vi "FRC3005_GyroXRS450_SPI_Accumulator_Loop.vi"(8 "error in":errorcluster, 10 "History Length (ms)":i32=2000, 11 "GyroDeviceRef":T1={"DevStatus"={"status"=FALSE, "code"=0, "source"=""}, "Analog Channel"=enum."AI 0", "Offset"=0.0, "Gain (VoltsPerDegree/Second)"=0.0, "Gyro Type"=enum."Analog", "Handle"=0, "SPI Bus"=enum."Invalid", "Device Found"=FALSE, "Sample Rate"=1.0, "Calibrate On Open"=FALSE} {"Sample Rate" min=0.25 max=100.0 step=0.25}) -> (0 "error out":errorcluster)   [LabVIEW 2016, in "Path Track.lvlib"]
doc: "Periodically reads the SimpleGyro and makes data available to your robot project. Place this block within PeriodicTasks.vi."
uses:
  Path Track.lvlib
  <vilib>/Rock Robotics/WPI/Gyro/WPI_GyroDevRef.ctl
  <vilib>/Rock Robotics/SystemInterfaces/AI/FPGA_AIChannel.ctl
  <vilib>/Rock Robotics/SystemInterfaces/spilib/spi_bus.ctl
  <vilib>/Rock Robotics/WPI/SPI/WPI_SPIDevRef.ctl
  FGV Control.ctl
  <vilib>/Platform/TimedLoop/XDataNode/timing_clust.ctl
  <vilib>/Platform/TimedLoop/XDataNode/nitl_modes.ctl
  <vilib>/Platform/TimedLoop/XDataNode/wakeup.ctl
  <vilib>/Platform/TimedLoop/XDataNode/XDataNode.xnode
  <vilib>/Platform/TimedLoop/XDataNode/XDNodeRunTimeDep.lvlib
  <vilib>/ptbypt/NI_PtbyPt.lvlib
panel:
  out "Rate":dbl
  out "Device Found":bool
  out "Offset":dbl
  out "Angle":dbl
  # "Analog"
  # "XRS"
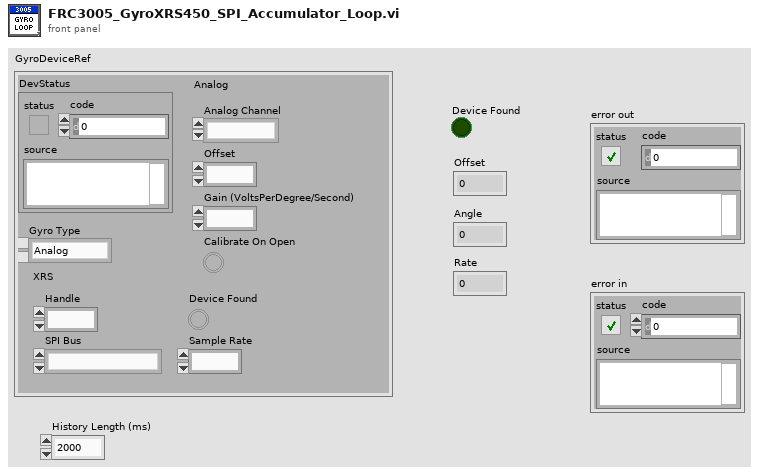
[diagram p1: front panel]
types:
  T1 = typedef "WPI_GyroDevRef.ctl" = cluster{"DevStatus":errorcluster, "Analog Channel":T2, "Offset":dbl, "Gain (VoltsPerDegree/Second)":dbl, "Gyro Type":enum16{"Analog", "XRS450"}, "Handle":i32, "SPI Bus":T3, "Device Found":bool, "Sample Rate":dbl, "Calibrate On Open":bool}
  T2 = typedef "FPGA_AIChannel.ctl" = enum8{"AI 0", "AI 1", "AI 2", "AI 3", "AI MXP 0", "AI MXP 1", "AI MXP 2", "AI MXP 3", "Invalid"}
  T3 = typedef "spi_bus.ctl" = enum16{"SPI On-Board, CS0", "SPI On-Board, CS1", "SPI On-Board, CS2", "SPI On-Board, CS3", "SPI MXP", "Invalid"}
  T4 = typedef "WPI_SPIDevRef.ctl" = cluster{"DevStatus":errorcluster, "Handle":i32, "SPI Bus":T3}
  T5 = typedef "Path Track.lvlib/FGV Control.ctl" = enum16{"Allocate", "Get", "Append"}
  T6 = typedef "XDNodeRunTimeDep.lvlib/timing_clust.ctl" = cluster{"Expected End [f-1]":u64, "Actual End [f-1]":u64, "Finished Late? [f-1]":bool, "Expected End [i-1]":u64, "Actual End [i-1]":u64, "Finished Late? [i-1]":bool, "Expected Start [i]":u64, "Actual Start [i]":u64, "Expected Start [f]":u64, "Actual Start [f]":u64, "Source Name":string, "Structure Name":string, "Period":i64, "Deadline":i64, "Offset":i64, "Start":i64, "Priority":i32, "Timeout":i32, "Mode":T7, "Wakeup Reason":T8, "Error":errorcluster, "Source Type":string, "Secondary Source Type":string, "Global End Time":u64, "Global Start Time":u64, "Frame Duration":u64, "Iteration Duration":u64, "Assigned CPU":i32, "I/O Scan Engine Mode":u32}
  T7 = typedef "XDNodeRunTimeDep.lvlib/nitl_modes.ctl" = enum32{"No Change", "Process missed periods, maintain original phase", "Discard missed periods, maintain original phase", "Process missed periods, ignore original phase", "Discard missed periods, ignore original phase"}
  T8 = typedef "XDNodeRunTimeDep.lvlib/wakeup.ctl" = enum32{"Normal", "Aborted", "Asynchronous wakeup", "Timing source error", "Timed loop error", "Timeout"}
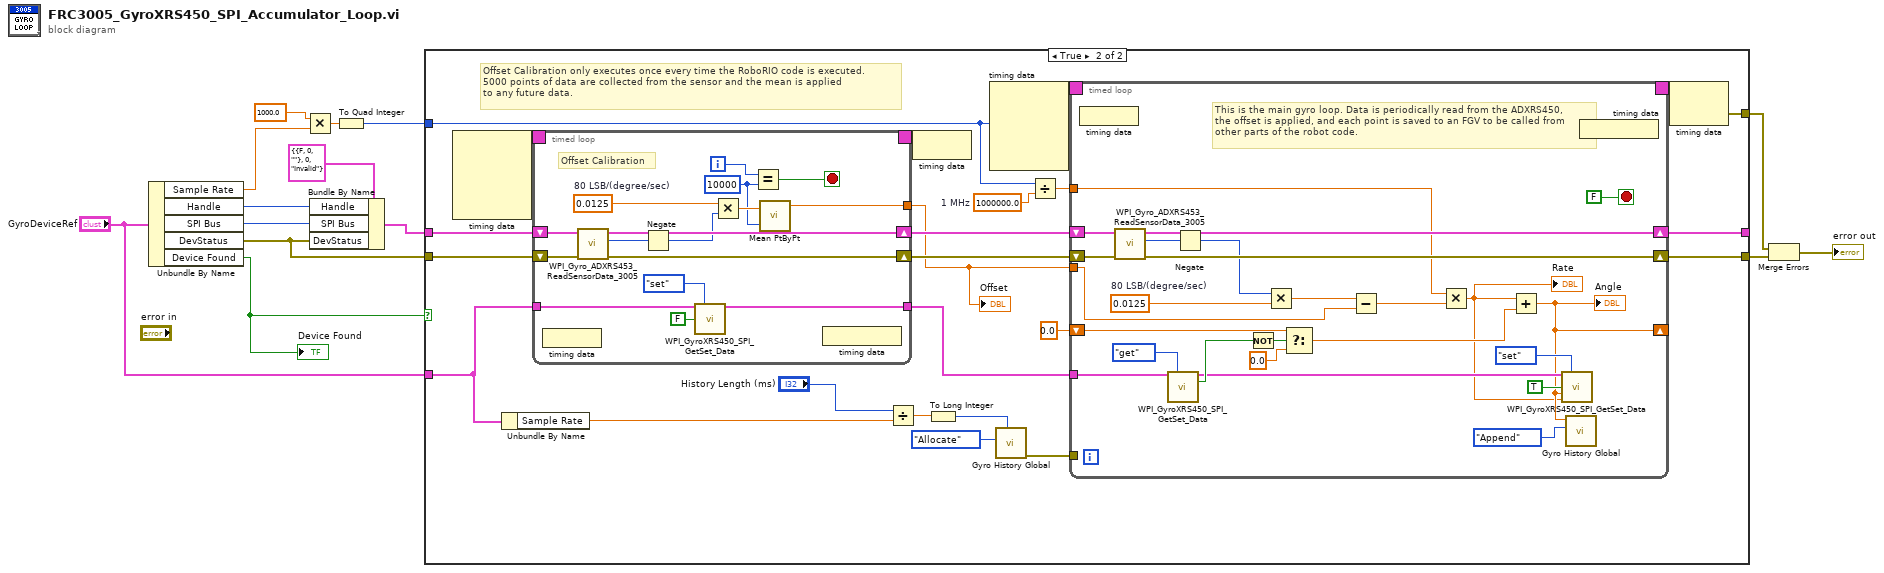
[diagram p0: block diagram]
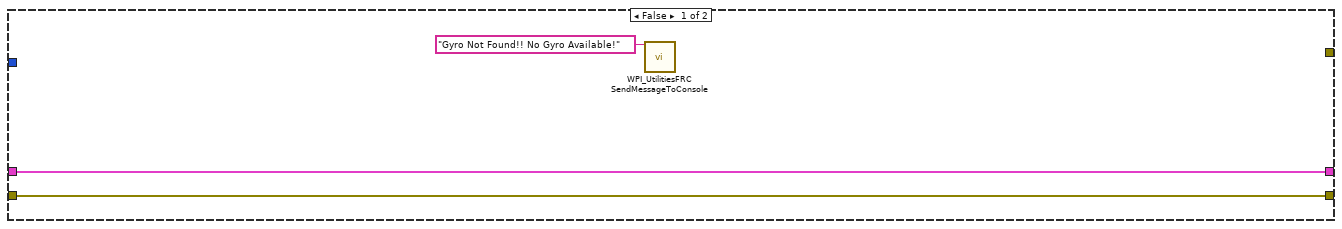
[diagram p2: hidden frame]
diagram:
  n1 = Unbundle By Name("GyroDeviceRef") -> ("Sample Rate"=w5:dbl, "Handle"=w14:i32, "SPI Bus"=w13:T3, "DevStatus"=w2:errorcluster, "Device Found"=w12:bool)
  "Device Found" <- w12
  n2 = Multiply(x=1000.0 ("y"), y=w5) -> (x*y=w11:dbl)
  n3 = Bundle By Name(cluster=T4 {"DevStatus"={"status"=FALSE, "code"=0, "source"=""}, "Handle"=0, "SPI Bus"=enum."Invalid"} ("SPIDevRef"), "Handle"=w14, "SPI Bus"=w13, "DevStatus"=w2) -> (w3:T4)
  n4 = To Quad Integer(1:w11) -> (0:w10:i64)
  n5 = case shown="True" w12 {
    tunnel: w3 -> [w17 w30]
    tunnel: w2 -> [w16 w29]
    tunnel: [w16 w39] -> w8
    tunnel: [w17 w38] -> _
    tunnel: w10 -> [_ w36]
    tunnel: "GyroDeviceRef" -> [_ w24]
    tunnel: [_ w35] -> w7
    frame False {
      n6 = call <vilib>:"WPI_UtilitiesFRC SendMessageToConsole.vi"("Message"="Gyro Not Found!! No Gyro Available!") -> ()  [unwired: 14 in, 1 out]
    }
    frame True {
      w33 = 1000000.0  # 1 MHz
      # "Offset Calibration only executes once every time the RoboRIO code is executed.\n5000 points of data are collected from the sensor and the mean is applied\nto any future data."
      n7 = node-c288() -> (w32:T6)  [unwired: 4 in]
      n8 = Unbundle By Name(w24) -> ("Sample Rate"=w23:dbl)
      n9 = timed-loop {
        shift-right: [w55] -> w28
        shift-left: w30 -> [w57]
        shift-right: [w52] -> w27
        shift-left: w29 -> [w56]
        timing: w32 -> [_]
        timing-out: [_] -> w31
        tunnel: [w50] -> w26
        tunnel: w24 -> [w43]
        tunnel: [w44] -> w25
        i -> [w49]
        stop <- w47 stop-if-true
        w48 = 10000 ("y")
        w53 = 0.0125  # 80 LSB/(degree/sec)
        # "Offset Calibration"
        n10 = node-c288() -> ()  [unwired: 1 in]
        n11 = call "WPI_Gyro_ADXRS453_ReadSensorData_3005.vi"("error in (no error)"=w56, "SPIDevRef in"=w57) -> ("error out"=w52:errorcluster, "Sensor Data (n-1)"=w54:i16, "SPIDevRef out"=w55:T4)  [unwired: 5 in, 2 out]
        n12 = Negate(x=w54) -> (-x=w42:i16)
        n13 = call <vilib>:"WPI_GyroXRS450_SPI_GetSet_Data.vi"("GyroDeviceRef"=w43, "Operation"=enum16{"set", "get"}."set", "Calibrated"=FALSE) -> ("GyroDeviceRef"=w44:T1)  [unwired: 8 in, 4 out]
        n14 = Multiply(x=w53, y=w42) -> (x*y=w51:dbl)
        n15 = Equal?(x=w49, y=w48) -> (x = y?=w47:bool)
        n16 = call <vilib>:"Mean PtByPt.vi"("x"=w51, "sample length"=w48) -> ("mean"=w50:dbl)  [unwired: 2 in, 1 out]
        n17 = node-c288() -> ()  [unwired: 1 out]
      }
      "Offset" <- w26
      n18 = Divide(x="History Length (ms)", y=w23) -> (x/y=w21:dbl)
      n19 = node-c288(w31) -> ()
      n20 = To Long Integer(number=w21) -> (32bit integer=w19:i32)
      n21 = node-c288(w36) -> (w41:T6)  [unwired: 3 in]
      n22 = call "Gyro History Global.vi"("Allocate Size"=w19, "Operation"=FGV_Control."Allocate") -> ("error out"=w18:errorcluster)  [unwired: 8 in, 1 out]
      n23 = Divide(x=w36, y=w33) -> (x/y=w37:dbl)
      n24 = timed-loop {
        shift-right: [w83] -> w38
        shift-left: w28 -> [w85]
        shift-right: [w79] -> w39
        shift-left: w27 -> [w84]
        timing: w41 -> [_]
        timing-out: [_] -> w40
        shift-right: [w63] -> _
        shift-left: 0.0 -> [w80]
        tunnel: w37 -> [w65]
        tunnel: w25 -> [w68]
        tunnel: w26 -> [w71]
        tunnel: w18 -> [_]
        stop <- FALSE stop-if-true
        w81 = 0.0125  # 80 LSB/(degree/sec)
        # "This is the main gyro loop. Data is periodically read from the ADXRS450, \nthe offset is applied, and each point is saved to an FGV to be called from\nother parts of the robot code."
        n25 = node-c288() -> ()  [unwired: 1 in]
        n26 = call "WPI_Gyro_ADXRS453_ReadSensorData_3005.vi"("error in (no error)"=w84, "SPIDevRef in"=w85) -> ("error out"=w79:errorcluster, "Sensor Data (n-1)"=w82:i16, "SPIDevRef out"=w83:T4)  [unwired: 5 in, 2 out]
        n27 = call <vilib>:"WPI_GyroXRS450_SPI_GetSet_Data.vi"("GyroDeviceRef"=w68, "Operation"=enum16{"set", "get"}."get") -> ("GyroDeviceRef"=w67:T1, "Reset?"=w73:bool)  [unwired: 9 in, 3 out]
        n28 = Negate(x=w82) -> (-x=w62:i16)
        n29 = Not(x=w73) -> (.not. x?=w76:bool)
        n30 = Multiply(x=w62, y=w81) -> (x*y=w72:dbl)
        n31 = Select(t=w80, s=w76, f=0.0 ("t")) -> (s? t:f=w78:dbl)
        n32 = Subtract(x=w72, y=w71) -> (x-y=w70:dbl)
        n33 = Multiply(x=w65, y=w70) -> (x*y=w61:dbl)
        "Rate" <- w61
        n34 = Add(x=w61, y=w78) -> (x+y=w63:dbl)
        "Angle" <- w63
        n35 = call <vilib>:"WPI_GyroXRS450_SPI_GetSet_Data.vi"("GyroDeviceRef"=w67, "Operation"=enum16{"set", "get"}."set", "Calibrated"=TRUE, "Angle"=w63, "Rate"=w61) -> ()  [unwired: 6 in, 5 out]
        n36 = call "Gyro History Global.vi"("Operation"=FGV_Control."Append", "Gyro"=w63) -> ()  [unwired: 8 in, 2 out]
        n37 = node-c288() -> ()  [unwired: 1 out]
      }
      n38 = node-c288(w40) -> (w35:errorcluster)
    }
  }
  n39 = Merge Errors(w7, w8) -> (→"error out":errorcluster)
